vi "InitializeRunInfoDatabase.vi"() -> ()   [LabVIEW 2014]
uses:
  <vilib>/addons/h5labview2/base/hclass_t.ctl
  <vilib>/addons/h5labview2/base/hid_t.ctl
  <vilib>/addons/h5labview2/file/H5Fmode.ctl
  <vilib>/addons/h5labview2/base/lib_path.vi
  <vilib>/addons/h5labview2/base/H5Equery.vi
  <vilib>/addons/h5labview2/dataset/H5Dwrite.llb/H5Dwrite.xnode
  <vilib>/addons/h5labview2/file/H5F.lvlib
  <vilib>/addons/h5labview2/dataset/H5D.lvlib
  <vilib>/addons/h5labview2/group/H5G.lvlib
panel:
  out "type out":T1 format="%.0x"
  out "class":T2
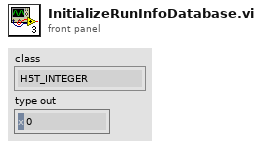
[diagram p1: front panel]
types:
  T1 = typedef "hid_t.ctl" = i32
  T2 = typedef "hclass_t.ctl" = enum16{"H5T_INTEGER", "H5T_FLOAT", "H5T_TIME", "H5T_STRING", "H5T_BITFIELD", "H5T_OPAQUE", "H5T_COMPOUND", "H5T_REFERENCE", "H5T_ENUM", "H5T_VLEN", "H5T_ARRAY"}
  T3 = cluster{"run_number":i32, "file_path":string, "LED_freq_Hz":dbl, "LED_pulse_width_ns":dbl, "multiplicity_requirement":u8, "HV_status":bool, "run_type":string, "comments":string, "material_in_tank":string, "start_time_UNIX":dbl, "start_time_string":string}
  T4 = typedef "H5F.lvlib/H5Fmode.ctl" = enum16{"read-only", "read-write", "overwrite", "create new", "open or create"}
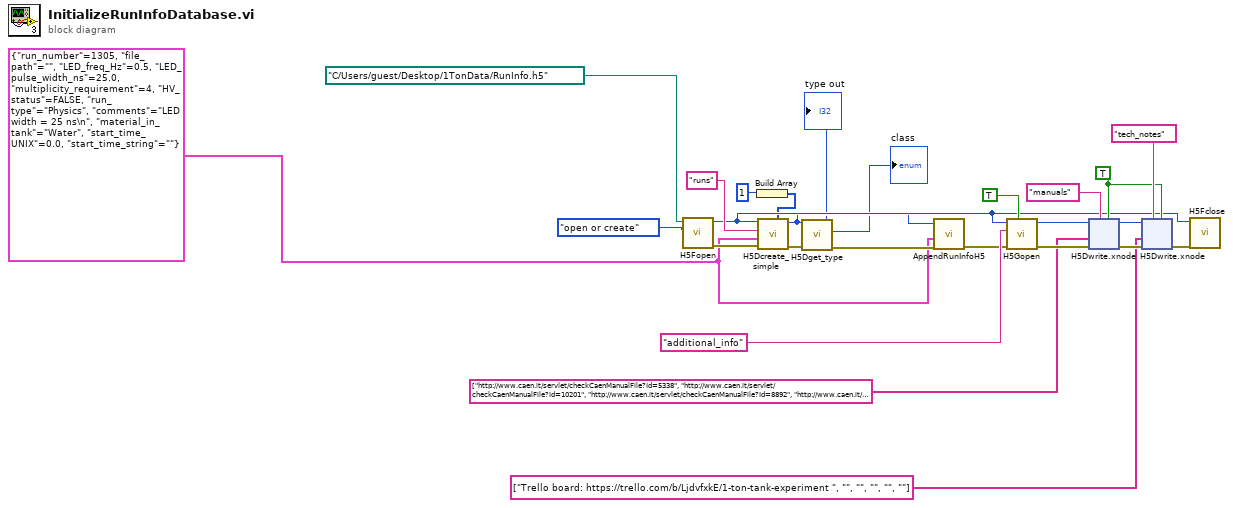
[diagram p0: block diagram]
diagram:
  w1 = T3 {"run_number"=1305, "file_path"="", "LED_freq_Hz"=0.5, "LED_pulse_width_ns"=25.0, "multiplicity_requirement"=4, "HV_status"=FALSE, "run_type"="Physics", "comments"="LED width = 25 ns\n", "material_in_tank"="Water", "start_time_UNIX"=0.0, "start_time_string"=""} ("Cluster")
  w14 = TRUE ("replace? (F)")
  n1 = call <vilib>:"H5Fopen.vi"("mode (read-only)"=H5Fmode."open or create", "path"=path "C:/Users/guest/Desktop/1TonData/RunInfo.h5") -> ("error out"=w24:errorcluster, "ref out"=w10:T1)  [unwired: 8 in]
  n2 = Build Array(1 ("ndims")) -> (w3:i32[])
  n3 = call <vilib>:"H5Dcreate_simple.vi"("chunk size"=w3, "error in (no error)"=w24, "type in"=w1, "name"="runs", "ref in"=w10) -> ("error out"=w8:errorcluster, "dset out"=w7:T1)  [unwired: 5 in]
  n4 = call <vilib>:"H5Dget_type.vi"("error in (no error)"=w8, "ref in"=w7) -> ("error out"=w6:errorcluster, "class"=→"class":T2, "type out"=→"type out":T1)  [unwired: 7 in]
  n5 = call "AppendRunInfoH5.vi"("error in (no error)"=w6, "RunInfo"=w1, "dset in"=w7) -> ("error out"=w9:errorcluster)  [unwired: 8 in]
  n6 = call <vilib>:"H5Gopen.vi"("create? (F)"=TRUE, "error in (no error)"=w9, "name"="additional_info", "ref in"=w10) -> ("error out"=w18:errorcluster, "group out"=w19:T1)  [unwired: 6 in]
  n7 = xnode "H5Dwrite.xnode"("replace? (F)"=w14, "dataset name"="manuals", "error in (no error)"=w18, "data"=string[] ["http://www.caen.it/servlet/checkCaenManualFile?Id=5338", "http://www.caen.it/servlet/checkCaenManualFile?Id=10201", "http://www.caen.it/servlet/checkCaenManualFile?Id=8892", "http://www.caen.it/servlet/checkCaenManualFile?Id=5281", "http://www.caen.it/servlet/checkCaenManualFile?Id=5333", "http://www.caen.it/servlet/checkCaenManualFile?Id=5465"], "ref in"=w19) -> ("error out"=w17:errorcluster, "ref out"=w16:i32)  [unwired: 2 in, 1 out]
  n8 = xnode "H5Dwrite.xnode"("replace? (F)"=w14, "dataset name"="tech_notes", "error in (no error)"=w17, "data"=string[] ["Trello board: https://trello.com/b/LjdvfxkE/1-ton-tank-experiment ", "", "", "", "", ""], "ref in"=w16) -> ("error out"=w11:errorcluster)  [unwired: 2 in, 2 out]
  n9 = call <vilib>:"H5Fclose.vi"("error in (no error)"=w11, "ref"=w10) -> ()  [unwired: 9 in, 1 out]
